vi "FrontPanel.vi"() -> ()   [LabVIEW 2013]
uses:
  field-global.vi
  I-AC-global.vi
  resistance-global.vi
  temp-global.vi
  stop-machine-global.vi
  IntegrationTime-global.vi
  Stop_B_Global.vi
  He3_Tlogger_Global 1.vi
  StopTempSweep.vi
panel:
  out "T Running":bool
  out "B Running":bool
  in  "Stop B Sweep":bool
  in  "Index2":i32
  in  "Index":i32
  in  "SAVE":bool
  in  "Path 2":path
  in  "Path":path
  in  "SAVE":bool
  in  "wait time /ms":u32=1000
  out "Resistance v Field":cluster{"Y":dbl[], "Y":dbl[]}[](graph)
  out "Resistance v Temp":cluster{"Y":dbl[], "Y":dbl[]}[](graph)
  in  "Points":i32=10
  in  "End Current /A":dbl=1.0
  in  "Start Current /A":dbl
  in  "Time Constant (8: 100ms) 2":u16(ring)=8 items=["10 us", "30 us", "100 us", "300 us", "1 ms", "3 ms", "10 ms", "30 ms", "100 ms", "300 ms", "1 s", "3 s", "10 s", "30 s", "100 s", "300 s", "1 ks", "3 ks", "10 ks", "30 ks"]
  out "Temperature":dbl[](graph)
  out "Device Resistance":dbl[](graph)
  out "Lock In Current":dbl[](graph)
  out "B FIeld":dbl[](graph)
  in  "stop":bool
  in  "Stop Temp Sweep":bool
  in  "Temperature Threshold":dbl=1.0
  in  "TSweep Start":bool
  in  "B Sweep Start":bool
  # "INTEGRATION CONSTANT"
  # "TEMPERATURE SWEEP"
  # "B-FIELD\nSWEEP"
  # "STOP ME FIRST!"
  # "STOP ME FIRST!"
  # "I Use Colons as\nFile Seperators"
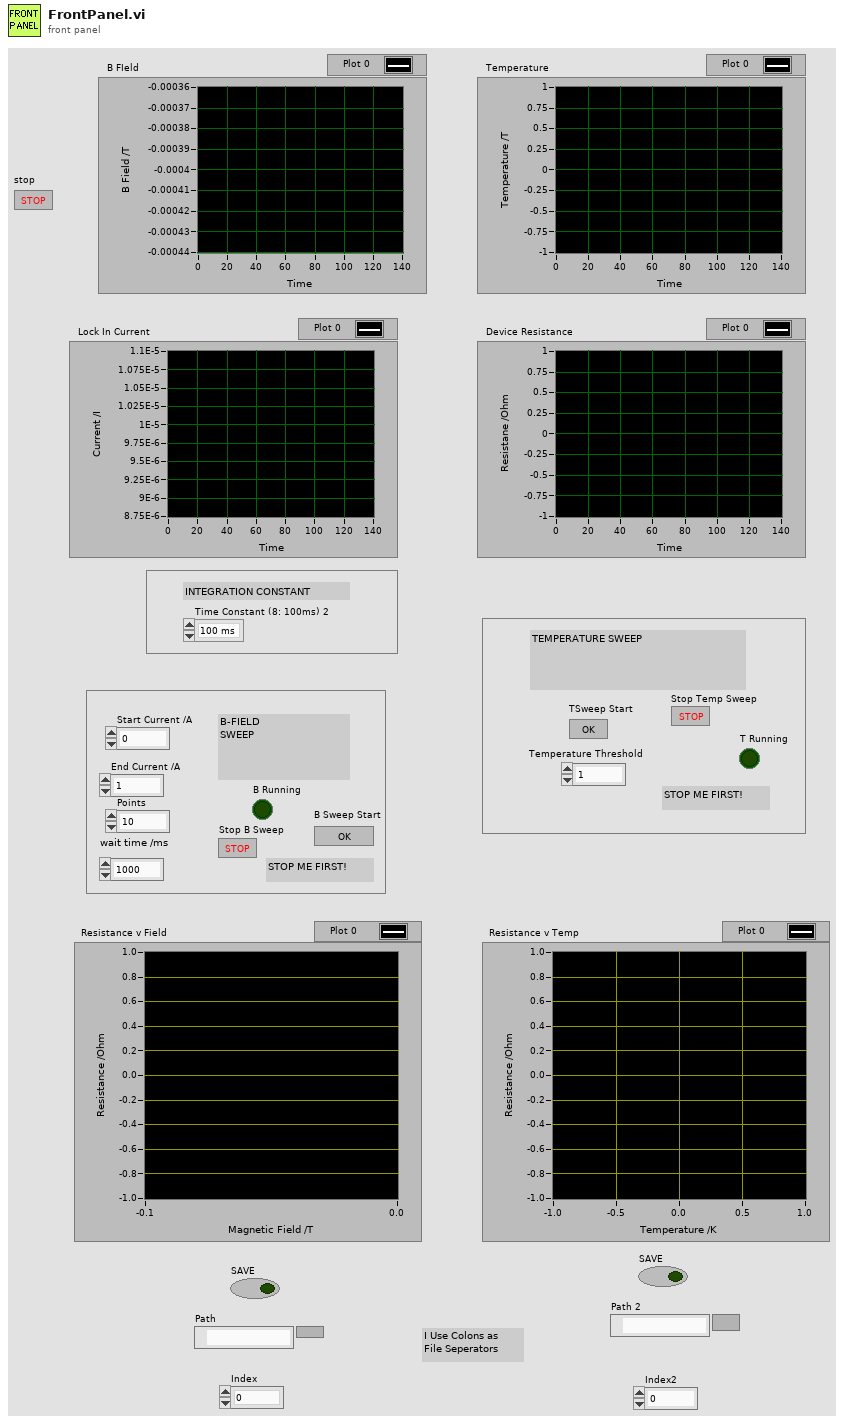
[diagram p1: front panel]
types:
  T1 = enum16{"Init", "Close", "Idle", "TSweep", "BSweep"}
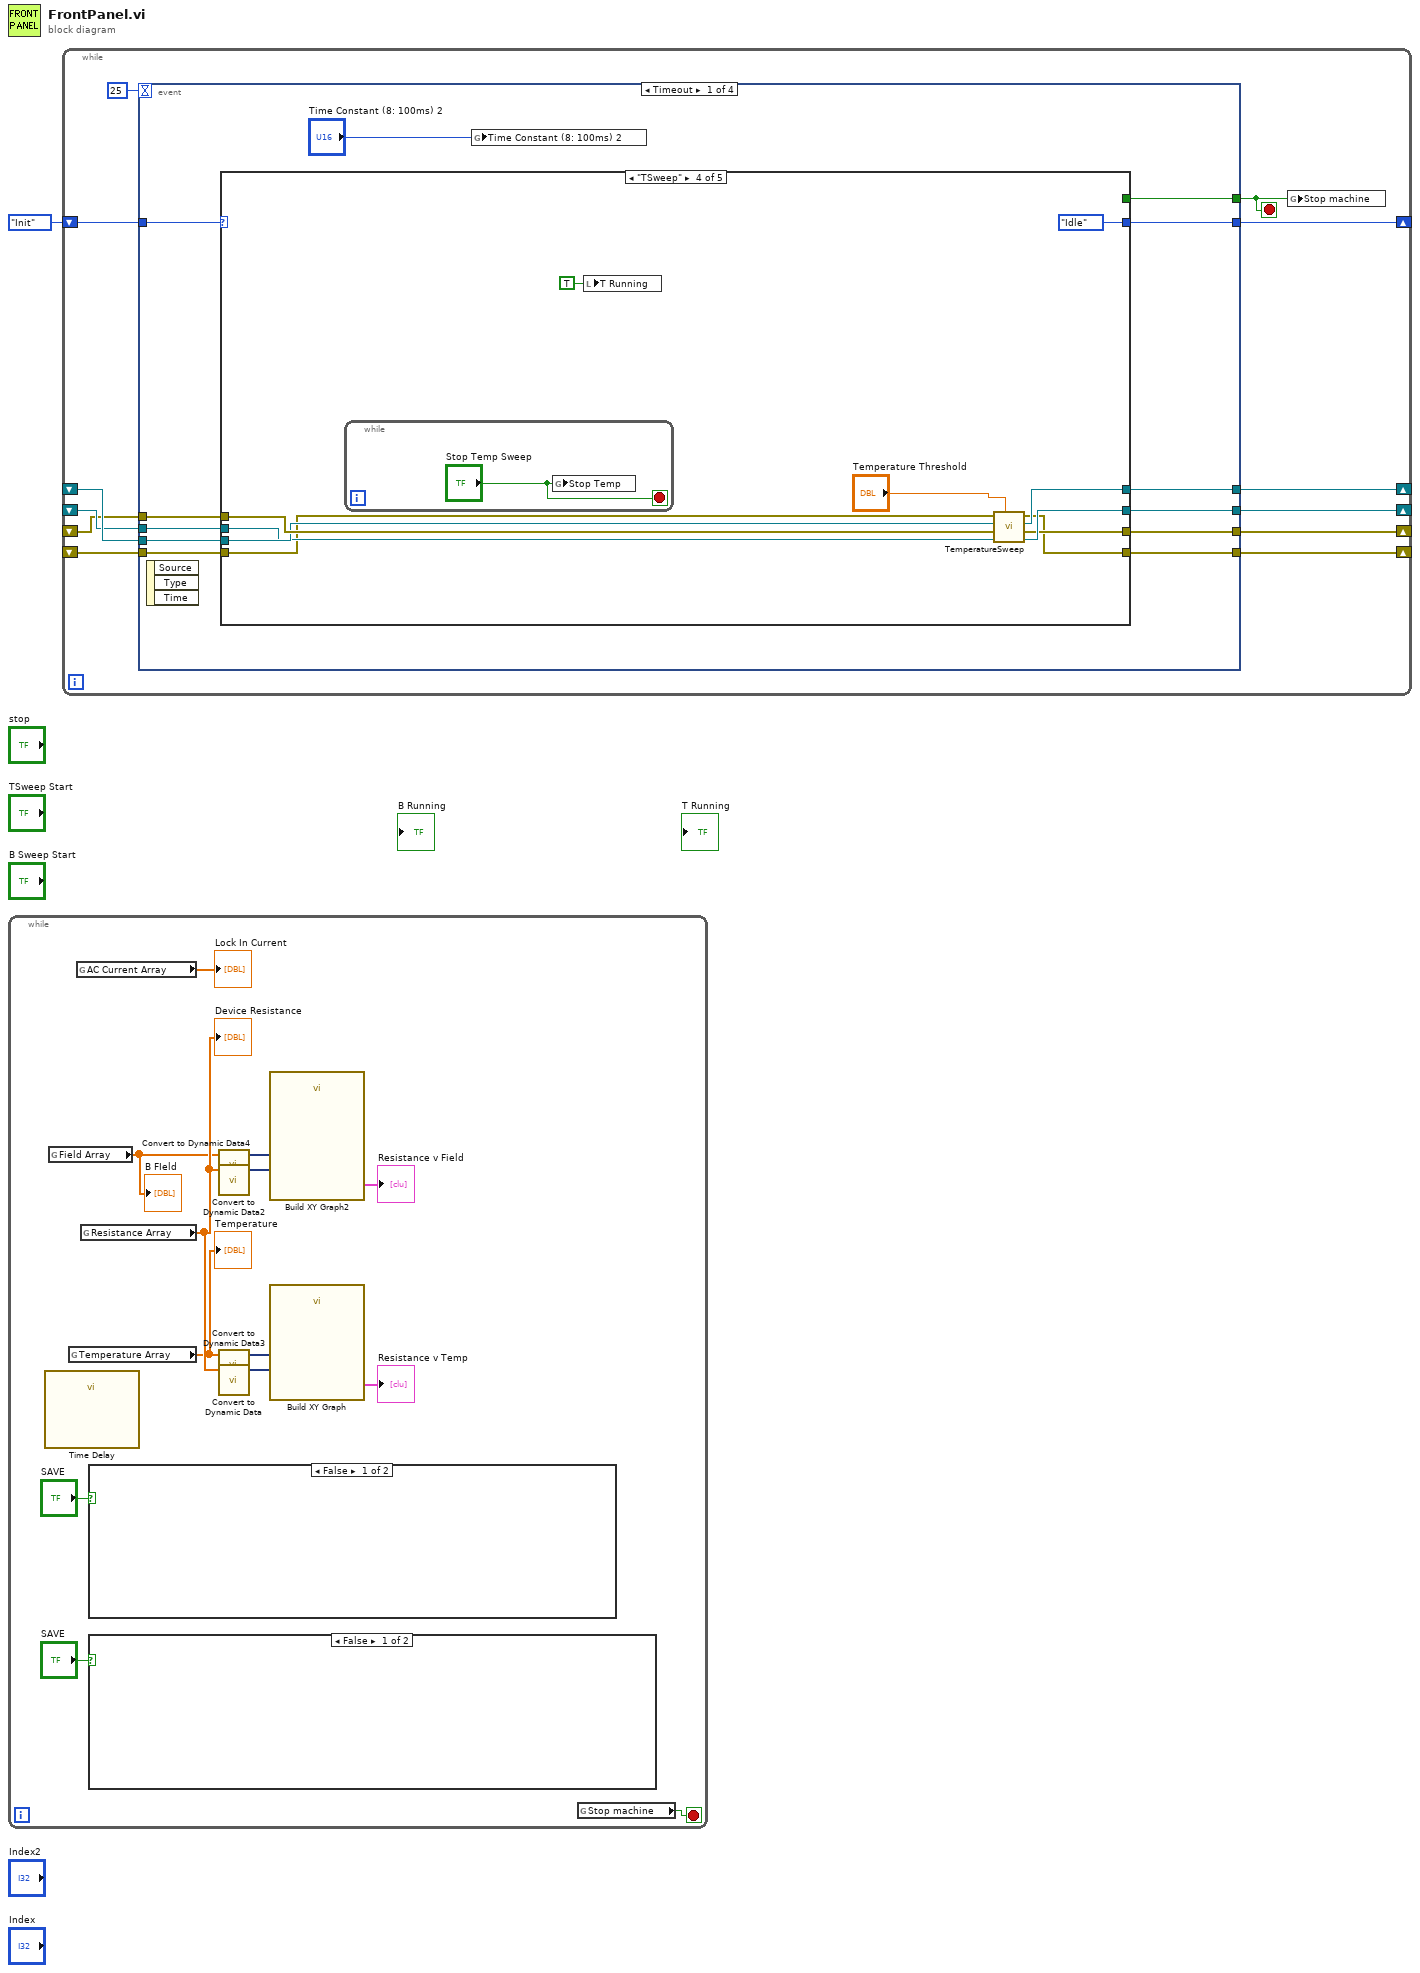
[diagram p0: block diagram]
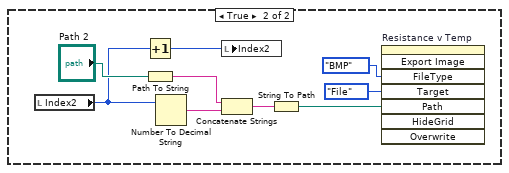
[diagram p2: hidden frame]
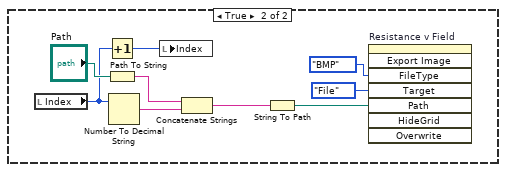
[diagram p3: hidden frame]
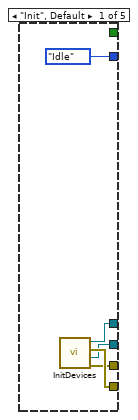
[diagram p4: hidden frame]
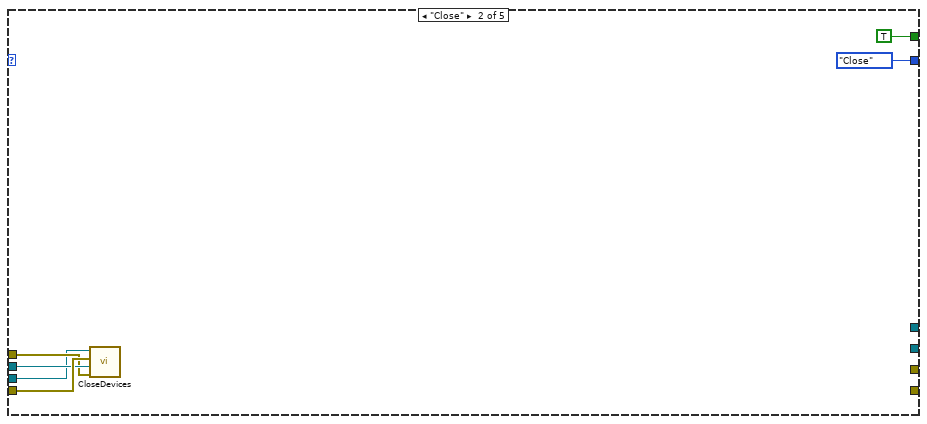
[diagram p5: hidden frame]
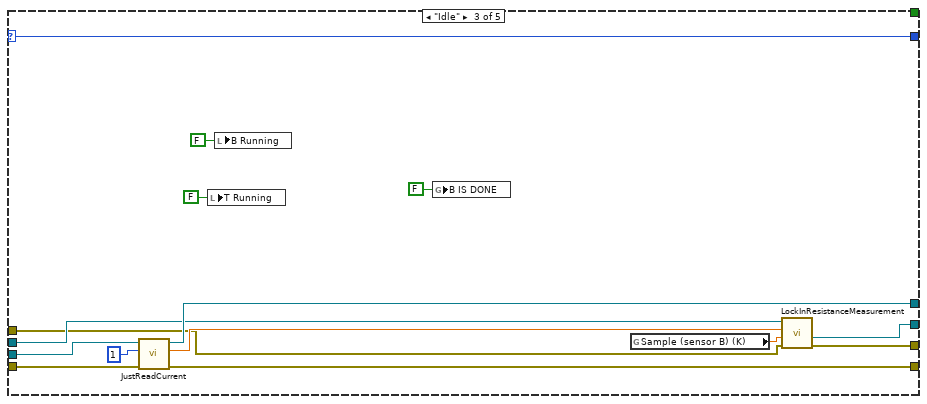
[diagram p6: hidden frame]
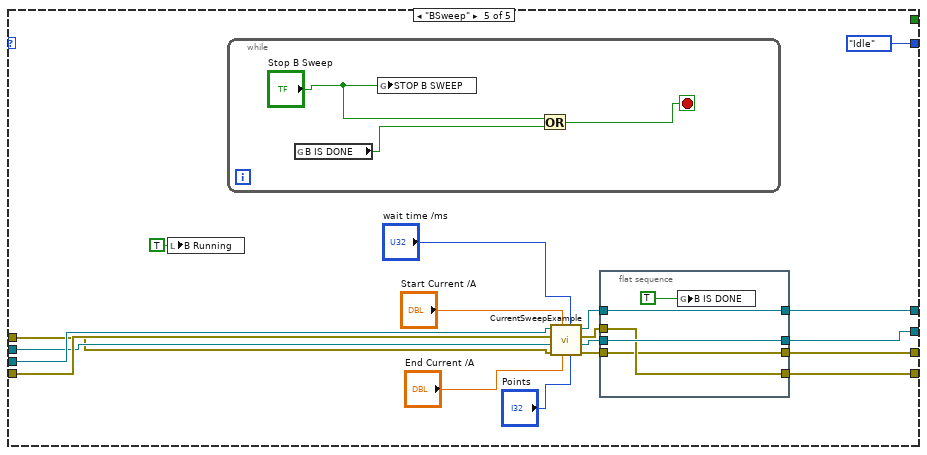
[diagram p7: hidden frame]
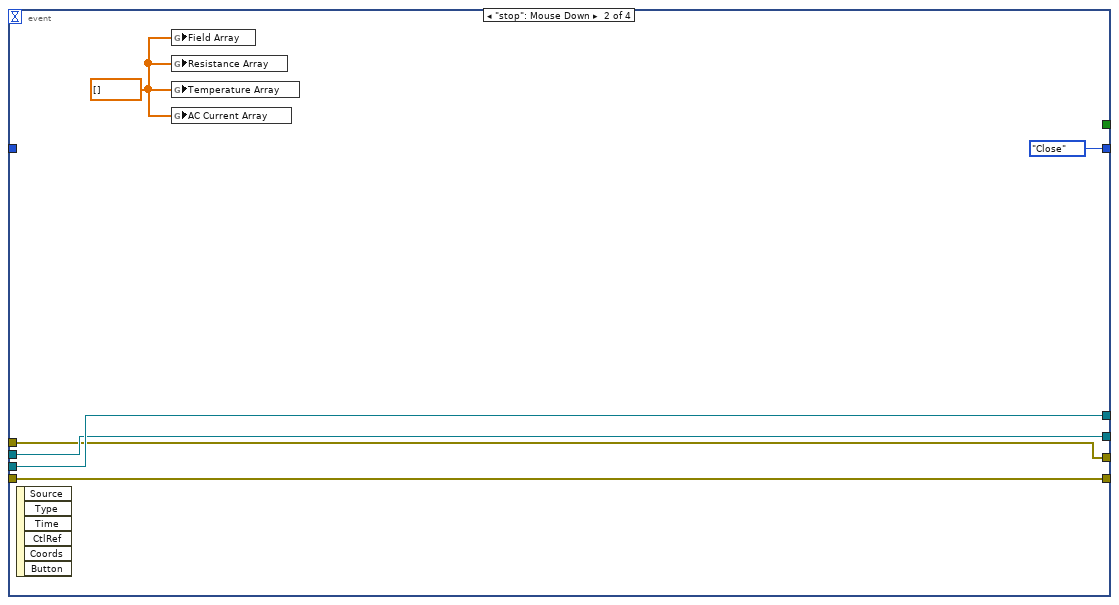
[diagram p8: hidden frame]
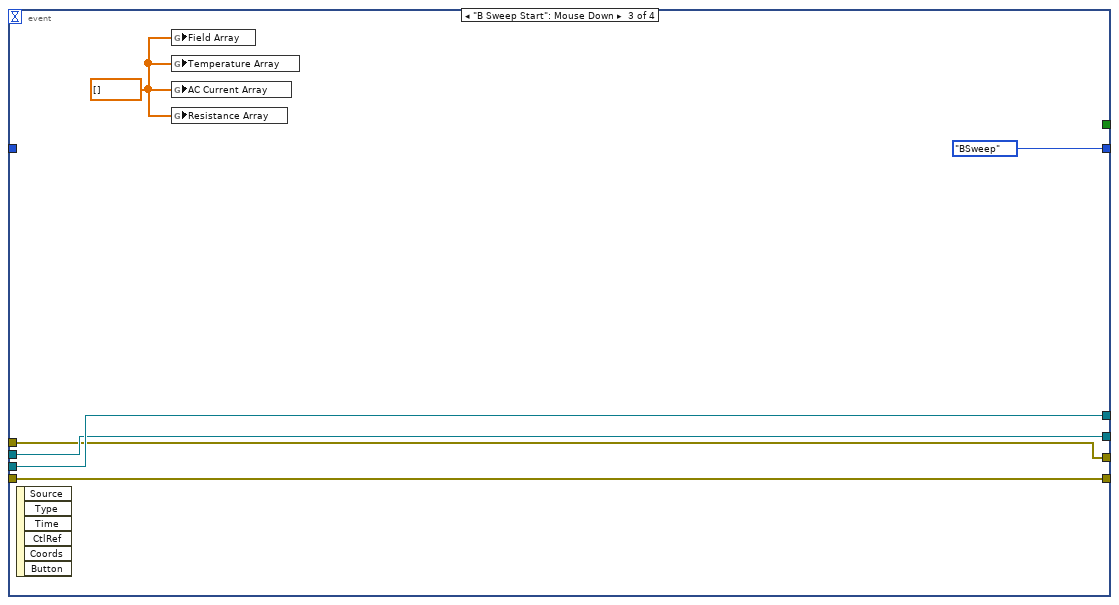
[diagram p9: hidden frame]
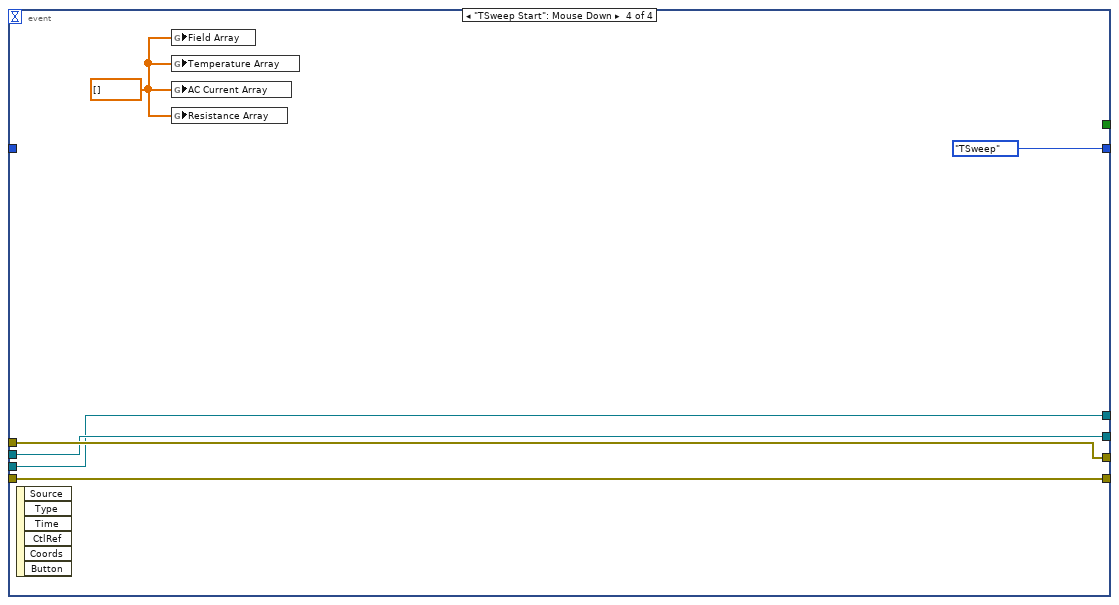
[diagram p10: hidden frame]
diagram:
  n1 = while {
    stop <- w14 stop-if-true
    n2 = call "Time Delay"() -> ()  [unwired: 11 in, 1 out]
    n3 = global read "field-global.vi" "Field Array"() -> (w5:dbl[])
    "B FIeld" <- w5
    n4 = global read "temp-global.vi" "Temperature Array"() -> (w7:dbl[])
    "Temperature" <- w7
    n5 = global read "I-AC-global.vi" "AC Current Array"() -> (→"Lock In Current":dbl[])
    n6 = global read "resistance-global.vi" "Resistance Array"() -> (w9:dbl[])
    "Device Resistance" <- w9
    n7 = case shown="False" "SAVE" {
      frame False {
      }
      frame True {
        n8 = local read "Index"() -> (w25:i32)
        n9 = Increment(x=w25) -> (x+1=w24:i32)
        n10 = Path To String(path="Path") -> (string=w29:string)
        n11 = Number To Decimal String(number=w25) -> (decimal integer string=w28:string)  [unwired: 1 in]
        n12 = local write "Index"(w24) -> ()
        n13 = Concatenate Strings(w29, w28) -> (w27:string)
        n14 = String To Path(string=w27) -> (path=w26:path)
        n15 = invoke on="Resistance v Field" class="XYGraph (strict)" method="Export Image"("FileType"=enum32{"BMP", "EPS", "EMF", "PICT"}."BMP" ("File Type"), "Target"=enum32{"File", "Clipboard"}."File", "Path"=w26) -> ()  [unwired: 5 in, 8 out]
      }
    }
    n16 = case shown="False" "SAVE" {
      frame False {
      }
      frame True {
        n17 = local read "Index2"() -> (w16:i32)
        n18 = Increment(x=w16) -> (x+1=w15:i32)
        n19 = Path To String(path="Path 2") -> (string=w20:string)
        n20 = Number To Decimal String(number=w16) -> (decimal integer string=w17:string)  [unwired: 1 in]
        n21 = local write "Index2"(w15) -> ()
        n22 = Concatenate Strings(w20, w17) -> (w19:string)
        n23 = String To Path(string=w19) -> (path=w18:path)
        n24 = invoke on="Resistance v Temp" class="XYGraph (strict)" method="Export Image"("FileType"=enum32{"BMP", "EPS", "EMF", "PICT"}."BMP" ("File Type"), "Target"=enum32{"File", "Clipboard"}."File", "Path"=w18) -> ()  [unwired: 5 in, 8 out]
      }
    }
    n25 = call "Convert to Dynamic Data4"("Array"=w5) -> ("Dynamic Data Type"=w4:dynamicdata)  [unwired: 3 in]
    n26 = call "Convert to Dynamic Data2"("Array"=w9) -> ("Dynamic Data Type"=w8:dynamicdata)  [unwired: 3 in]
    n27 = call "Convert to Dynamic Data3"("Array"=w7) -> ("Dynamic Data Type"=w6:dynamicdata)  [unwired: 3 in]
    n28 = call "Convert to Dynamic Data"("Array"=w9) -> ("Dynamic Data Type"=w10:dynamicdata)  [unwired: 3 in]
    n29 = call "Build XY Graph2"("Y Input"=w8, "X Input"=w4) -> ("XY Graph"=→"Resistance v Field":cluster{"X":dbl[], "Y":dbl[]}[])  [unwired: 8 in, 1 out]
    n30 = call "Build XY Graph"("Y Input"=w10, "X Input"=w6) -> ("XY Graph"=→"Resistance v Temp":cluster{"X":dbl[], "Y":dbl[]}[])  [unwired: 8 in, 1 out]
    n31 = global read "stop-machine-global.vi" "Stop machine"() -> (w14:bool)
  }
  n32 = while {
    shift-right: [w35] -> _
    shift-left: T1."Init" -> [w44]
    shift-right: [w43] -> _
    shift-left: _ -> [w39]
    shift-right: [w42] -> _
    shift-left: _ -> [w38]
    shift-right: [w41] -> _
    shift-left: _ -> [w37]
    shift-right: [w40] -> _
    shift-left: _ -> [w36]
    stop <- w33 stop-if-true
    n33 = event shown="[0] Timeout" {
      selector: _ -> [_ _ _ _]
      dyn-events: _ -> [_ _ _ _]
      timeout: 25 -> [_ _ _ _]
      tunnel: w44 -> [w56 _ _ _]
      tunnel: [w55 w125 w131 w134] -> w43
      tunnel: [w54 w122 w130 w135] -> w42
      tunnel: [w53 w124 w129 w136] -> w41
      tunnel: [w52 w123 w128 w137] -> w40
      tunnel: w39 -> [w51 w125 w131 w134]
      tunnel: w38 -> [w50 w122 w130 w135]
      tunnel: w37 -> [w49 w124 w129 w136]
      tunnel: w36 -> [w48 w123 w128 w137]
      tunnel: [w47 T1."Close" T1."BSweep" T1."TSweep"] -> w35
      tunnel: [w46 _ _ _] -> w33
      event Timeout {
        n34 = event-data() -> ()  [unwired: 1 in, 3 out]
        n35 = case shown="\"TSweep\"" w56 {
          selector: w56 -> [_ _ w82 _ _]
          tunnel: [w61 _ w80 w87 w102] -> w55
          tunnel: [w60 _ w79 w86 w98] -> w54
          tunnel: [w59 _ w71 w89 w100] -> w53
          tunnel: [w58 _ w72 w88 w96] -> w52
          tunnel: w51 -> [_ w62 w81 w91 w107]
          tunnel: w50 -> [_ w66 w78 w85 w106]
          tunnel: w49 -> [_ w65 w74 w90 w105]
          tunnel: w48 -> [_ w64 w73 w92 w104]
          tunnel: [T1."Idle" T1."Close" w82 T1."Idle" T1."Idle"] -> w47
          tunnel: [_ TRUE _ _ _] -> w46
          frame "Init", Default {
            n36 = call "InitDevices.vi"() -> ("Stanford Err"=w58:errorcluster, "Stanford ID"=w59:refnum<visa-resource-name>, "Keithley Err"=w60:errorcluster, "Keithley ID"=w61:refnum<visa-resource-name>)  [unwired: 8 in]
          }
          frame "Close" {
            n37 = call "CloseDevices.vi"("Stanford Err"=w64, "Stanford ID"=w65, "Keithley Err"=w66, "Keithley"=w62) -> ()  [unwired: 8 in]
          }
          frame "Idle" {
            n38 = call "JustReadCurrent.vi"("error in (no error)"=w78, "Function (0: Volts)"=u16 1, "Keithley In"=w81) -> ("error out"=w79:errorcluster, "Measured Current"=w76:dbl, "Keithley Out"=w80:refnum<visa-resource-name>)  [unwired: 6 in]
            n39 = local write "T Running"(FALSE ("T Running")) -> ()
            n40 = local write "B Running"(FALSE ("B Running")) -> ()
            n41 = global write "Stop_B_Global.vi" "B IS DONE"(FALSE ("B IS DONE")) -> ()
            n42 = global read "He3_Tlogger_Global 1.vi" "Sample (sensor B) (K)"() -> (w75:dbl)
            n43 = call "LockInResistanceMeasurement.vi"("Stanford Error In"=w73, "Temperature"=w75, "Keithley Current"=w76, "Stanford ID"=w74) -> ("error out"=w72:errorcluster, "Stanford ID"=w71:refnum<visa-resource-name>)  [unwired: 3 in, 2 out]
          }
          frame "TSweep" {
            n44 = while {
              stop <- "Stop Temp Sweep" stop-if-true
              n45 = global write "StopTempSweep.vi" "Stop Temp"("Stop Temp Sweep") -> ()
            }
            n46 = local write "T Running"(TRUE ("T Running")) -> ()
            n47 = call "TemperatureSweep.vi"("Threshold"="Temperature Threshold", "Stanford In"=w90, "Stanford Error"=w92, "Keithley In"=w91, "Keithley Error"=w85) -> ("Stanford Out"=w89:refnum<visa-resource-name>, "Stanford Err Out"=w88:errorcluster, "Keithley Out"=w87:refnum<visa-resource-name>, "Keithley Err Out"=w86:errorcluster)  [unwired: 3 in]
          }
          frame "BSweep" {
            n48 = local write "B Running"(TRUE ("Boolean")) -> ()
            n49 = while {
              stop <- w118 stop-if-true
              n50 = global read "Stop_B_Global.vi" "B IS DONE"() -> (w119:bool)
              n51 = global write "Stop_B_Global.vi" "STOP B SWEEP"("Stop B Sweep") -> ()
              n52 = Or(x="Stop B Sweep", y=w119) -> (x .or. y?=w118:bool)
            }
            n53 = call "CurrentSweepExample.vi"("Points"="Points", "milliseconds to wait"="wait time /ms", "End Current"="End Current /A", "Start Current"="Start Current /A", "Stanford Err"=w104, "Stanford"=w105, "Keithley Err"=w106, "Keithley"=w107) -> ("Stanford Err Out"=w97:errorcluster, "Stanford Out"=w101:refnum<visa-resource-name>, "Keithley Err Out"=w99:errorcluster, "Keithley Out"=w103:refnum<visa-resource-name>)
            n54 = flat-sequence {
              tunnel: w103 -> [w116]
              tunnel: [w116] -> w102
              tunnel: w101 -> [w115]
              tunnel: [w115] -> w100
              tunnel: w99 -> [w114]
              tunnel: [w114] -> w98
              tunnel: w97 -> [w113]
              tunnel: [w113] -> w96
              frame #0 {
                n55 = global write "Stop_B_Global.vi" "B IS DONE"(TRUE ("STOP B SWEEP")) -> ()
              }
            }
          }
        }
        n56 = global write "IntegrationTime-global.vi" "Time Constant (8: 100ms) 2"("Time Constant (8: 100ms) 2") -> ()
      }
      event "stop": Mouse Down {
        w121 = dbl[] []
        n57 = event-data() -> ()  [unwired: 1 in, 6 out]
        n58 = global write "field-global.vi" "Field Array"(w121) -> ()
        n59 = global write "resistance-global.vi" "Resistance Array"(w121) -> ()
        n60 = global write "temp-global.vi" "Temperature Array"(w121) -> ()
        n61 = global write "I-AC-global.vi" "AC Current Array"(w121) -> ()
      }
      event "B Sweep Start": Mouse Down {
        w127 = dbl[] []
        n62 = event-data() -> ()  [unwired: 1 in, 6 out]
        n63 = global write "field-global.vi" "Field Array"(w127) -> ()
        n64 = global write "temp-global.vi" "Temperature Array"(w127) -> ()
        n65 = global write "I-AC-global.vi" "AC Current Array"(w127) -> ()
        n66 = global write "resistance-global.vi" "Resistance Array"(w127) -> ()
      }
      event "TSweep Start": Mouse Down {
        w133 = dbl[] []
        n67 = event-data() -> ()  [unwired: 1 in, 6 out]
        n68 = global write "field-global.vi" "Field Array"(w133) -> ()
        n69 = global write "temp-global.vi" "Temperature Array"(w133) -> ()
        n70 = global write "I-AC-global.vi" "AC Current Array"(w133) -> ()
        n71 = global write "resistance-global.vi" "Resistance Array"(w133) -> ()
      }
    }
    n72 = global write "stop-machine-global.vi" "Stop machine"(w33) -> ()
  }
